vi "Check Current Row Status.vi"(1 "Row":i32, 2 "Active Positions":bool[](array[boolean]), 3 "Rack Status In":bool[](array[boolean])) -> (0 "Rack Status Out":bool[](array[boolean]))   [LabVIEW 2021]
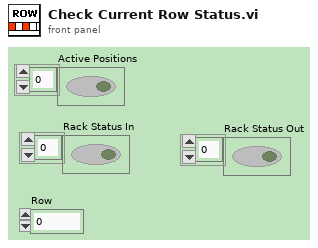
[diagram p1: front panel]
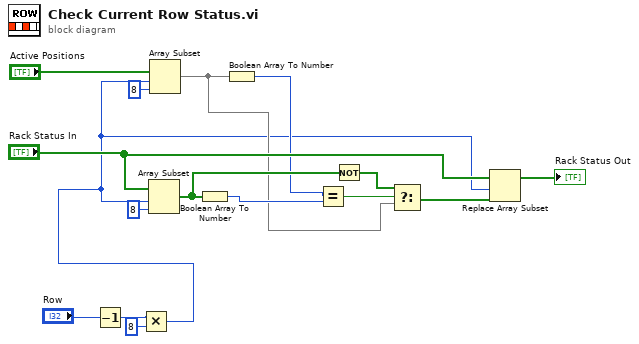
[diagram p0: block diagram]
diagram:
  n1 = Decrement(x="Row") -> (x-1=w9:i32)
  n2 = Multiply(x=w9, y=8) -> (x*y=w1:i32)
  n3 = Array Subset(array="Rack Status In", index=w1, length=8) -> (w12:bool[])
  n4 = Array Subset(array="Active Positions", index=w1, length=8) -> (w2:bool[])
  n5 = Boolean Array To Number(Boolean array=w12) -> (number=w6:u32)
  n6 = Boolean Array To Number(Boolean array=w2) -> (number=w5:u32)
  n7 = Equal?(x=w5, y=w6) -> (x = y?=w7:bool)
  n8 = Not(x=w12) -> (.not. x?=w13:bool[])
  n9 = Select(t=w13, s=w7, f=w2) -> (s? t:f=w14:bool[])
  n10 = Replace Array Subset(array="Rack Status In", new element=w14, index=w1) -> (→"Rack Status Out":bool[])
